vi "FixationInROI.vi"(2 "ROI rect":T1, 3 "ROI Type":dbl, 4 "old picture":picture, 5 "Fixations Array":dbl[][](array[numeric])) -> (0 "Fixations in ROI":dbl format="%.2f", 1 "new picture":picture)   [LabVIEW 2013]
uses:
  <vilib>/Analysis/baseanly.llb/Real Dot Product.vi
  <vilib>/Analysis/NI_AALBase.lvlib
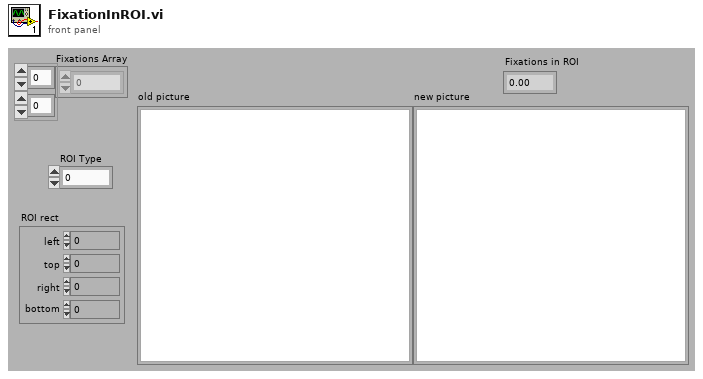
[diagram p1: front panel]
types:
  T1 = cluster{"left":i16, "top":i16, "right":i16, "bottom":i16}
  T2 = typedef "imagedata.ctl" = cluster{"image type":i32, "image depth":i32, "image":u8[], "mask":u8[], "colors":u32[], "Rectangle":cluster{"left":i16, "top":i16, "right":i16, "bottom":i16}}
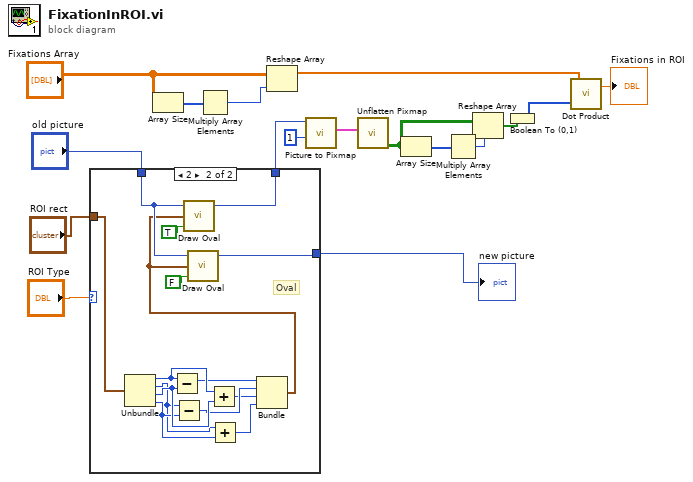
[diagram p0: block diagram]
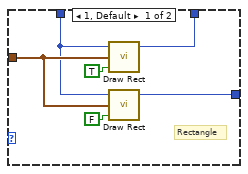
[diagram p2: hidden frame]
diagram:
  n1 = case shown="2" "ROI Type" {
    tunnel: "ROI rect" -> [w20 w33]
    tunnel: "old picture" -> [w19 w35]
    tunnel: [w23 w38] -> w3
    tunnel: [w18 w34] -> w2
    frame 1, Default {
      # "Rectangle"
      n2 = call <vilib>:"Draw Rect.vi"("picture"=w19, "rect"=w20, "fill?(F)"=TRUE) -> ("new picture"=w23:picture)  [unwired: 6 in]
      n3 = call <vilib>:"Draw Rect.vi"("picture"=w19, "rect"=w20, "fill?(F)"=FALSE) -> ("new picture"=w18:picture)  [unwired: 6 in]
    }
    frame 2 {
      # "Oval"
      n4 = Unbundle(w33) -> ("left"=w32:i16, "top"=w29:i16, "right"=w31:i16, "bottom"=w30:i16)
      n5 = Subtract(x=w32, y=w31) -> (x-y=w28:i16)
      n6 = Subtract(x=w29, y=w30) -> (x-y=w27:i16)
      n7 = Add(x=w32, y=w31) -> (x+y=w26:i16)
      n8 = Add(x=w29, y=w30) -> (x+y=w25:i16)
      n9 = Bundle(w28, w27, w26, w25) -> (w24:cluster{i16, i16, i16, i16})  [unwired: 1 in]
      n10 = call <vilib>:"Draw Oval.vi"("picture"=w35, "rect"=w24, "fill?(F)"=TRUE) -> ("new picture"=w38:picture)  [unwired: 6 in]
      n11 = call <vilib>:"Draw Oval.vi"("picture"=w35, "rect"=w24, "fill?(F)"=FALSE) -> ("new picture"=w34:picture)  [unwired: 6 in]
    }
  }
  "new picture" <- w2
  n12 = Array Size(array="Fixations Array") -> (size(s)=w14:i32[])
  n13 = Multiply Array Elements(1:w14) -> (0:w13:i32)
  n14 = Reshape Array("Fixations Array", w13) -> (w10:dbl[])
  n15 = call <vilib>:"Picture to Pixmap.vi"("depth"=1, "picture"=w3) -> ("image data"=w15:T2)  [unwired: 8 in, 1 out]
  n16 = call <vilib>:"Unflatten Pixmap.vi"("image data"=w15) -> ("1-bit pixmap"=w7:bool[][])  [unwired: 4 in, 6 out]
  n17 = Array Size(array=w7) -> (size(s)=w12:i32[])
  n18 = Multiply Array Elements(1:w12) -> (0:w11:i32)
  n19 = Reshape Array(w7, w11) -> (w6:bool[])
  n20 = Boolean To (0,1)(Boolean=w6) -> (0, 1=w5:i16[])
  n21 = call-poly <vilib>:"Dot Product.vi"("Y Vector"=w5, "X Vector"=w10) -> ("X * Y"=→"Fixations in ROI":dbl)  [unwired: 1 out]
